vi "APU + Event Timing v6 four shots.vi"() -> ()   [LabVIEW 2015]
uses:
  IP Source/APU/Input.ctl
  IP Source/APU/Output.ctl
  IP Source/APU/Settings.ctl
  IP Source/ECU Event/Timing/Capture Output.ctl
  IP Source/ECU Event/Timing/Measure Settings.ctl
  IP Source/Version Token.ctl
  IP Source/ECU Event/Timing/Measure Output.ctl
  IP Source/APU/Shared Settings.ctl
  <vilib>/Platform/TimedLoop/XDataNode/timing_clust.ctl
  <vilib>/Platform/TimedLoop/XDataNode/nitl_modes.ctl
  <vilib>/Platform/TimedLoop/XDataNode/wakeup.ctl
  IP Source/ECU Event/Timing/Capture Settings.ctl
  <vilib>/rvi/Emulation/niFpgaSctlEmulationGetInTimedLoop.vi
  <vilib>/rvi/Emulation/niFpgaEmulationReportErrorSimple.vi
  <vilib>/rvi/Emulation/niFpgaGetClockAttributes.vi
  <vilib>/rvi/Emulation/niFpgaCriticalErrorInLSC.vi
  <vilib>/rvi/eio/common/nirviEmuTemplateMethod_errors.vi
  IP Source/ECU Event/Timing/Measure Events (40MHz).vi
  <vilib>/Platform/TimedLoop/XDataNode/XDataNode.xnode
  <vilib>/eio/EIONode/EIONode.xnode
  <vilib>/Platform/TimedLoop/XDataNode/XDNodeRunTimeDep.lvlib
  IP Source/ECU Event/Timing/ECU Event Timing.lvlib
  IP Source/APU/APU.lvlib
  IP Source/Engine Simulation Toolkit.lvlib
panel:
  in  "shared settings.my apu":T1 {"start" format="%#.15g"}
  in  "go.my apu":bool
  out "measure output.spark 4":T2
  out "measure output.spark 5":T2
  out "measure output.spark 6":T2
  out "measure output.fi 6":T2
  out "measure output.fi 5":T2
  out "measure output.fi 4":T2
  out "measure output.fi 3":T2
  out "measure output.spark 3":T2
  out "measure output.spark 2":T2
  out "measure output.spark 1":T2
  out "measure output.fi 2":T2
  out "measure output.fi 1":T2
  in  "est.version":T3
  out "Output.spark 6 shot 1":T4
  out "Output.spark 1 shot 1":T4
  out "Output.spark 2 shot 1":T4
  out "Output.spark 3 shot 1":T4
  out "Output.spark 4 shot 1":T4
  out "Output.spark 5 shot 1":T4
  out "Output.spark 6 shot 2":T4
  out "Output.spark 1 shot 2":T4
  out "Output.spark 2 shot 2":T4
  out "Output.spark 3 shot 2":T4
  out "Output.spark 4 shot 2":T4
  out "Output.spark 5 shot 2":T4
  out "Output.spark 6 shot 3":T4
  out "Output.spark 1 shot 3":T4
  out "Output.spark 2 shot 3":T4
  out "Output.spark 3 shot 3":T4
  out "Output.spark 4 shot 3":T4
  out "Output.spark 5 shot 3":T4
  out "Output.spark 6 shot 4":T4
  out "Output.spark 1 shot 4":T4
  out "Output.spark 2 shot 4":T4
  out "Output.spark 3 shot 4":T4
  out "Output.spark 4 shot 4":T4
  out "Output.spark 5 shot 4":T4
  in  "Settings.spark 1":T5
  in  "Settings.spark 2":T5
  in  "Settings.spark 3":T5
  in  "Settings.spark 4":T5
  in  "Settings.spark 5":T5
  in  "Settings.spark 6":T5
  in  "Settings.fi 6":T5
  in  "Settings.fi 5":T5
  in  "Settings.fi 4":T5
  in  "Settings.fi 3":T5
  in  "Settings.fi 2":T5
  in  "Settings.fi 1":T5
  out "Output.fi 6 shot 4":T4
  out "Output.fi 1 shot 4":T4
  out "Output.fi 2 shot 4":T4
  out "Output.fi 3 shot 4":T4
  out "Output.fi 4 shot 4":T4
  out "Output.fi 5 shot 4":T4
  out "Output.fi 6 shot 3":T4
  out "Output.fi 1 shot 3":T4
  out "Output.fi 2 shot 3":T4
  out "Output.fi 3 shot 3":T4
  out "Output.fi 4 shot 3":T4
  out "Output.fi 5 shot 3":T4
  out "Output.fi 6 shot 2":T4
  out "Output.fi 1 shot 2":T4
  out "Output.fi 2 shot 2":T4
  out "Output.fi 3 shot 2":T4
  out "Output.fi 4 shot 2":T4
  out "Output.fi 5 shot 2":T4
  out "Output.fi 5 shot 1":T4
  out "Output.fi 4 shot 1":T4
  out "Output.fi 3 shot 1":T4
  out "Output.fi 2 shot 1":T4
  out "Output.fi 1 shot 1":T4
  out "Output.fi 6 shot 1":T4
  in  "Settings.my apu":T6 caption="settings"
  out "Output.my apu":T7 caption="output"
  in  "Input.my apu":T8={"desired speed"=0.0, "reset"=TRUE} caption="input"
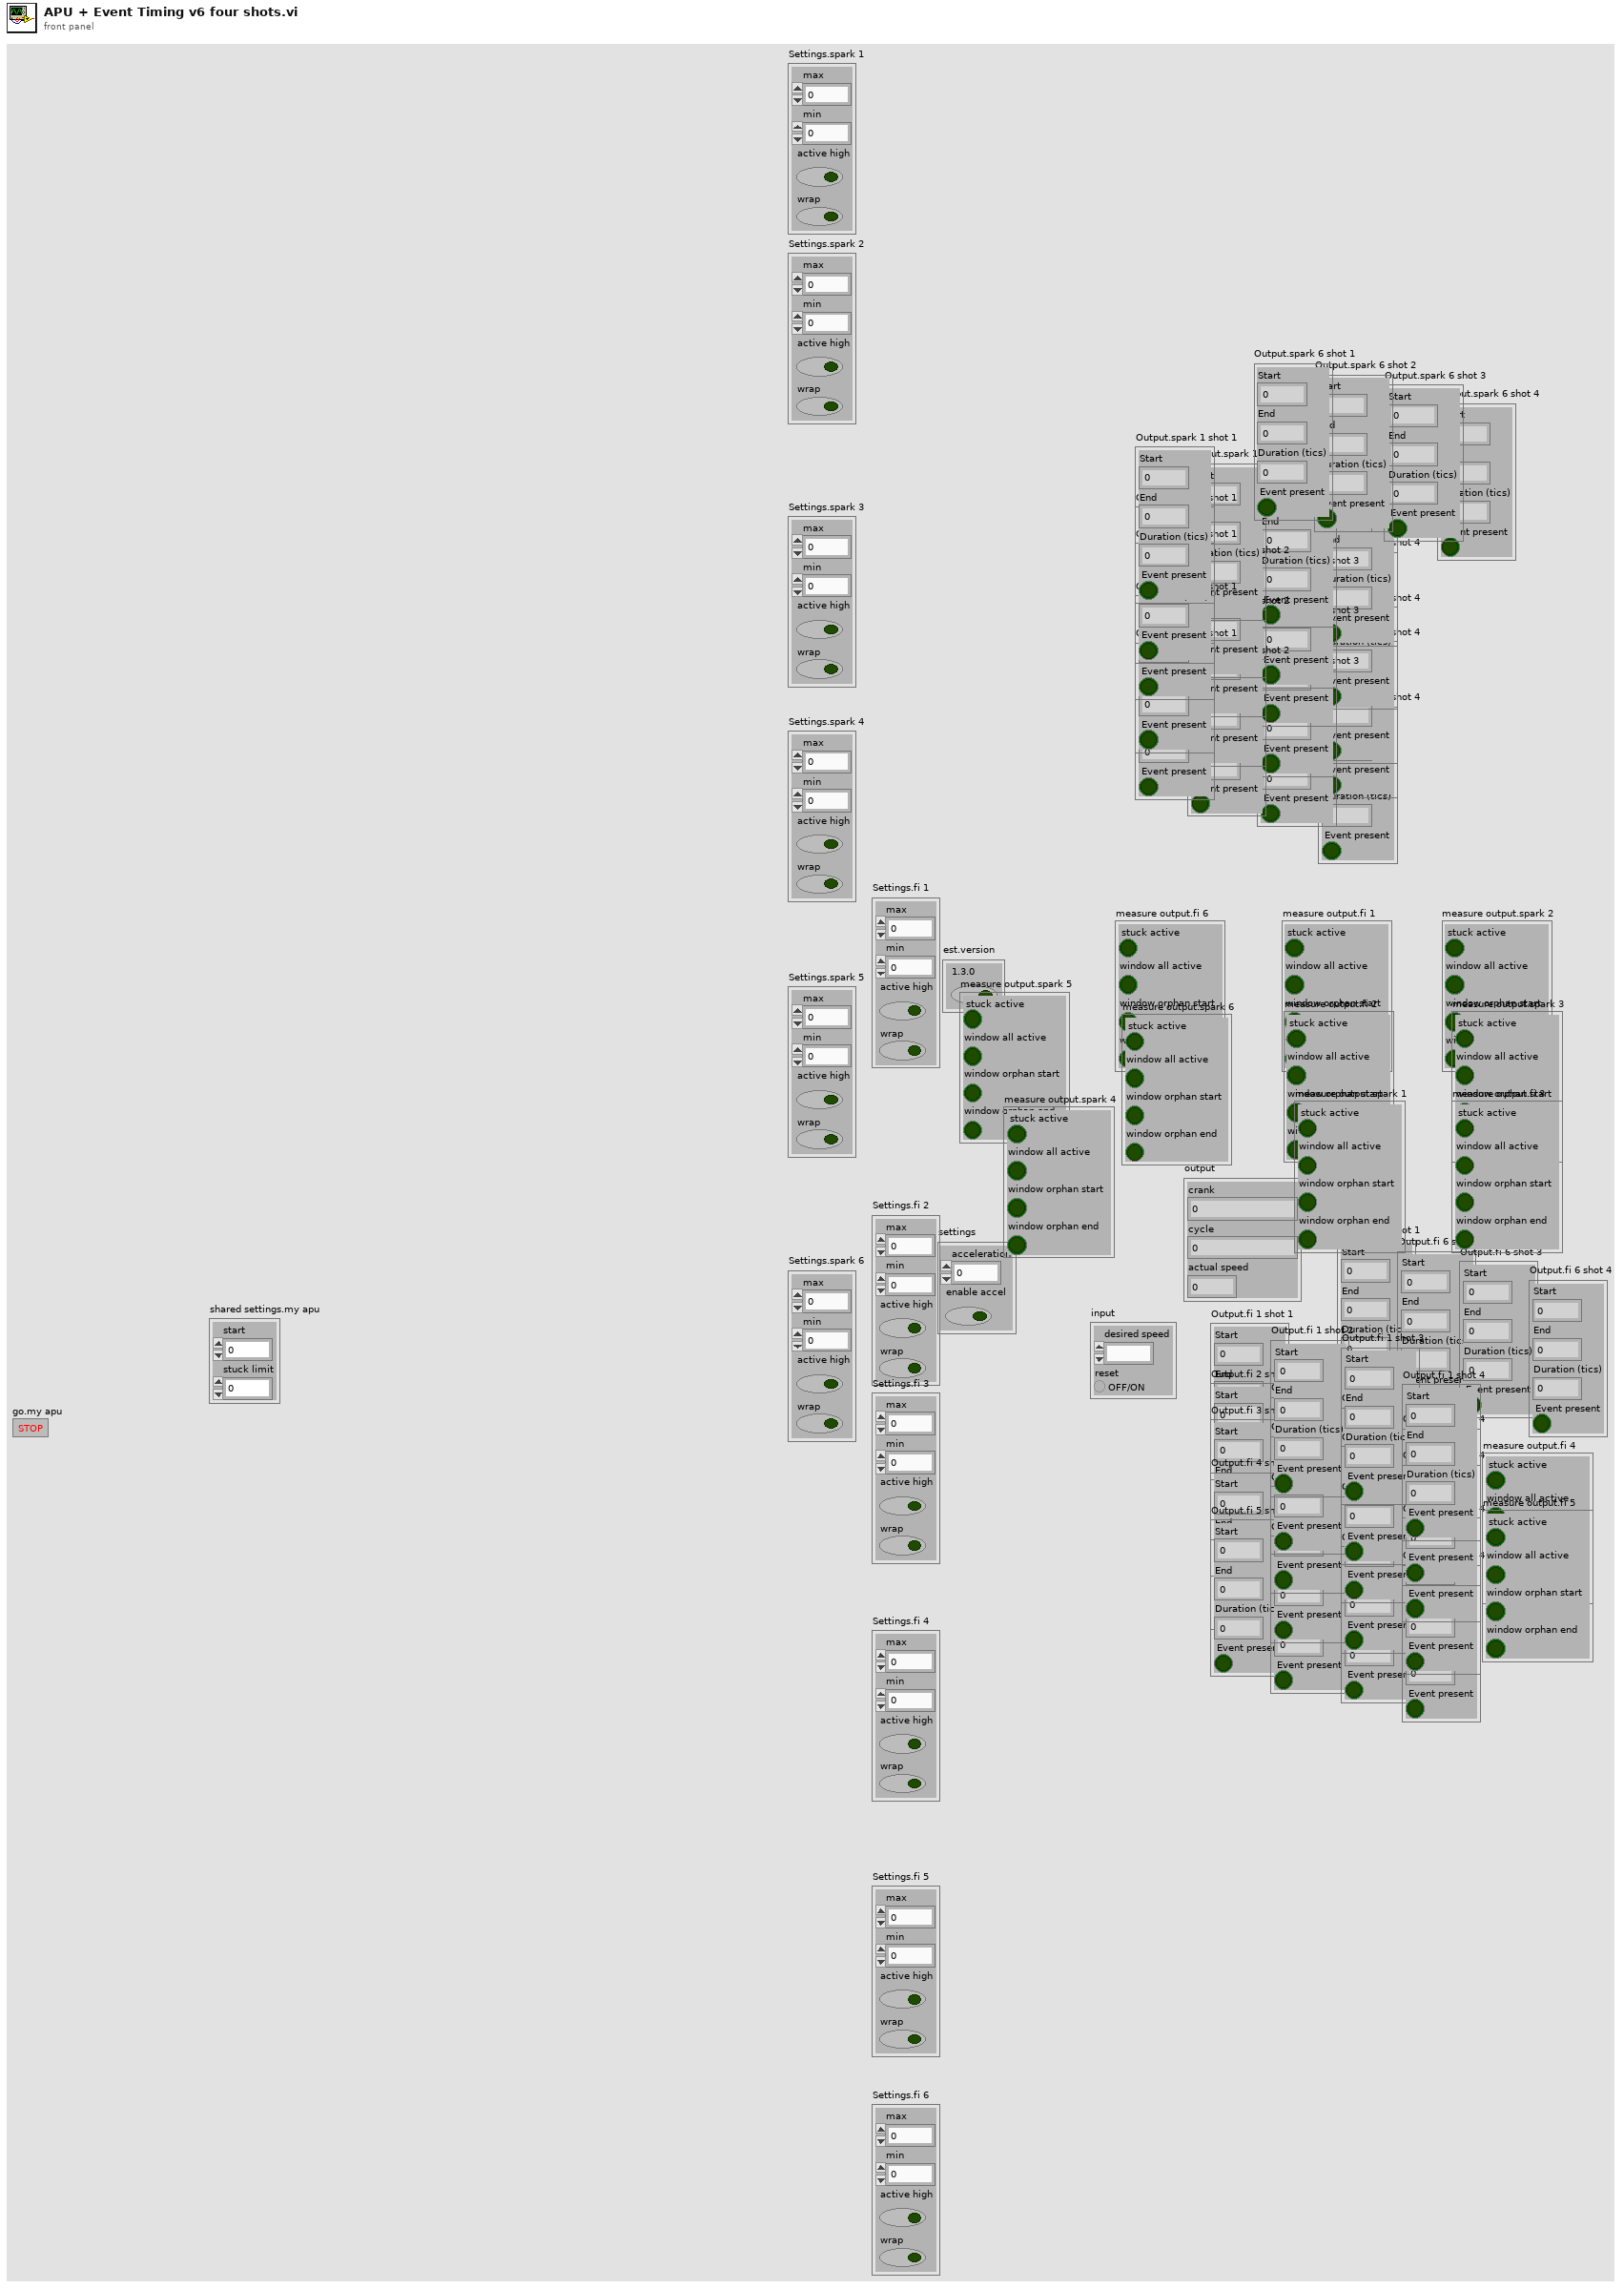
[diagram p1: front panel]
types:
  T1 = typedef "Engine Simulation Toolkit.lvlib/APU.lvlib/Shared Settings.ctl" = cluster{"start":fxp<+,17,17>, "stuck limit":fxp<+,18,18>}
  T2 = typedef "Engine Simulation Toolkit.lvlib/ECU Event Timing.lvlib/Measure Output.ctl" = cluster{"stuck active":bool, "window all active":bool, "window orphan start":bool, "window orphan end":bool}
  T3 = typedef "Engine Simulation Toolkit.lvlib/Version Token.ctl" = cluster{"1.3.0":bool}
  T4 = typedef "Engine Simulation Toolkit.lvlib/ECU Event Timing.lvlib/Capture Output.ctl" = cluster{"Start":u16, "End":u16, "Duration (tics)":fxp<+,18,18>, "Event present":bool}
  T5 = typedef "Engine Simulation Toolkit.lvlib/ECU Event Timing.lvlib/Measure Settings.ctl" = cluster{"max":u16, "min":u16, "active high":bool, "wrap":bool}
  T6 = typedef "Engine Simulation Toolkit.lvlib/APU.lvlib/Settings.ctl" = cluster{"acceleration":fxp<+,18,-20>, "enable accel":bool}
  T7 = typedef "Engine Simulation Toolkit.lvlib/APU.lvlib/Output.ctl" = cluster{"crank":u16, "cycle":u16, "actual speed":fxp<+/-,23,2>}
  T8 = typedef "Engine Simulation Toolkit.lvlib/APU.lvlib/Input.ctl" = cluster{"desired speed":fxp<+/-,23,2>, "reset":bool}
  T9 = typedef "XDNodeRunTimeDep.lvlib/timing_clust.ctl" = cluster{"Expected End [f-1]":u64, "Actual End [f-1]":u64, "Finished Late? [f-1]":bool, "Expected End [i-1]":u64, "Actual End [i-1]":u64, "Finished Late? [i-1]":bool, "Expected Start [i]":u64, "Actual Start [i]":u64, "Expected Start [f]":u64, "Actual Start [f]":u64, "Source Name":string, "Structure Name":string, "Period":i64, "Deadline":i64, "Offset":i64, "Start":i64, "Priority":i32, "Timeout":i32, "Mode":T10, "Wakeup Reason":T11, "Error":errorcluster, "Source Type":string, "Secondary Source Type":string, "Global End Time":u64, "Global Start Time":u64, "Frame Duration":u64, "Iteration Duration":u64, "Assigned CPU":i32, "I/O Scan Engine Mode":u32}
  T10 = typedef "XDNodeRunTimeDep.lvlib/nitl_modes.ctl" = enum32{"No Change", "Process missed periods, maintain original phase", "Discard missed periods, maintain original phase", "Process missed periods, ignore original phase", "Discard missed periods, ignore original phase"}
  T11 = typedef "XDNodeRunTimeDep.lvlib/wakeup.ctl" = enum32{"Normal", "Aborted", "Asynchronous wakeup", "Timing source error", "Timed loop error", "Timeout"}
  T12 = typedef "Engine Simulation Toolkit.lvlib/APU.lvlib/Register Bus.ctl" = cluster{"Speed":refnum<k21>, "Crank Angle":refnum<k21>, "Cycle Angle":refnum<k21>, "Crank Count":refnum<k21>, "Cycle Count":refnum<k21>, "1.25 MHz Counter":refnum<k21>, "Crank Rollover":refnum<k21>, "Cycle Rollover":refnum<k21>, "shared settings":T1}
  T13 = typedef "Engine Simulation Toolkit.lvlib/ECU Event Timing.lvlib/Capture Settings.ctl" = u8
  T14 = typedef "Engine Simulation Toolkit.lvlib/ECU Event Timing.lvlib/Measured Data.ctl" = cluster{"start":u16, "end":u16, "duration (tics)":fxp<+,18,18>, "window end":bool, "window begin":bool, "pulse end":bool, "pulse #":u8}
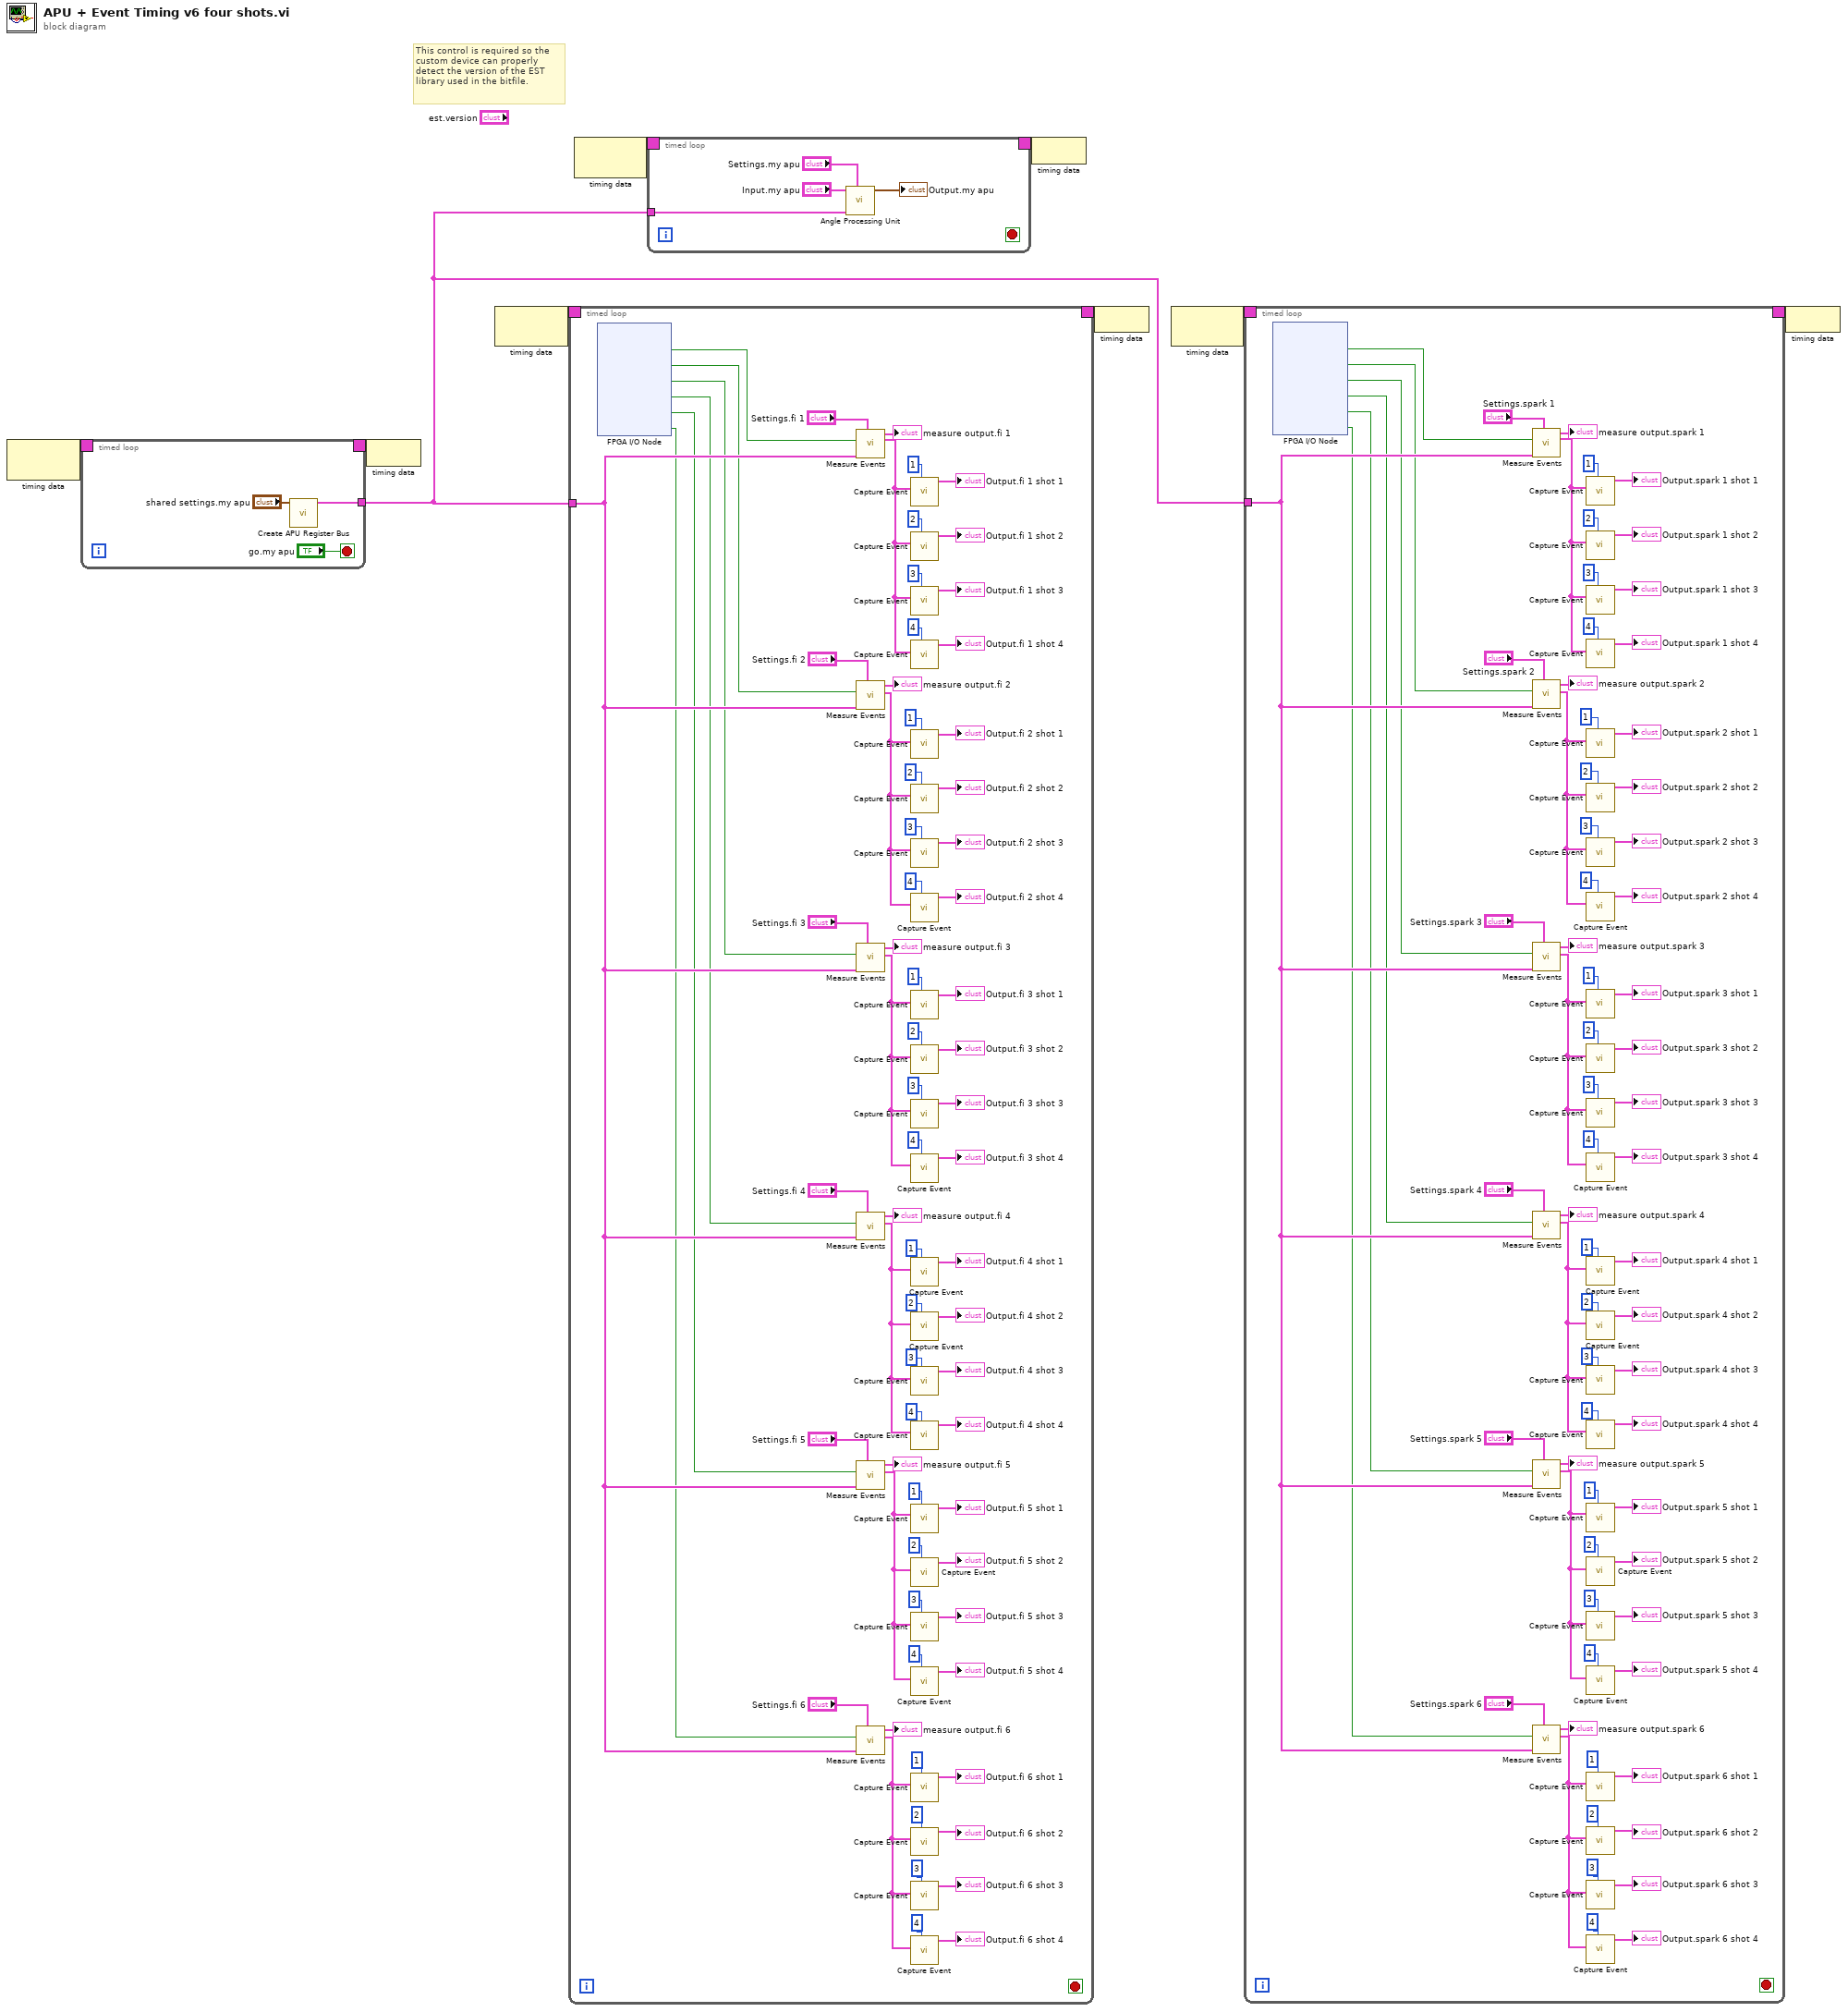
[diagram p0: block diagram]
diagram:
  # "This control is required so the custom device can properly detect the version of the EST library used in the bitfile."
  n1 = node-c288() -> (w3:T9)  [unwired: 1 in]
  n2 = timed-loop {
    timing: w3 -> [_]
    timing-out: [_] -> w2
    tunnel: [w12] -> w1
    stop <- "go.my apu" stop-if-true
    n3 = call "Create APU Register Bus.vi"("shared settings.<user name>"="shared settings.my apu") -> ("register bus"=w12:T12)  [unwired: 10 in]
  }
  n4 = node-c288(w2) -> ()
  n5 = node-c288() -> (w7:T9)  [unwired: 1 in]
  n6 = timed-loop {
    timing: w7 -> [_]
    timing-out: [_] -> w6
    tunnel: w1 -> [w63]
    stop <- _ stop-if-true
    n7 = xnode "FPGA I/O Node"() -> ("DIO0_0"=w56:bool, "DIO1_0"=w36:bool, "DIO2_0"=w35:bool, "DIO3_0"=w34:bool, "DIO4_0"=w22:bool, "DIO5_0"=w21:bool)  [unwired: 6 in, 6 out]
    n8 = call-poly "Measure Events.vi"("settings.<user name>"="Settings.fi 1", "register bus"=w63, "event"=w56) -> ("measured data"=w57:T14, "status.<user name>"=→"measure output.fi 1":T2)  [unwired: 7 in]
    n9 = call-poly "Measure Events.vi"("settings.<user name>"="Settings.fi 2", "register bus"=w63, "event"=w36) -> ("measured data"=w37:T14, "status.<user name>"=→"measure output.fi 2":T2)  [unwired: 7 in]
    n10 = call-poly "Measure Events.vi"("settings.<user name>"="Settings.fi 3", "register bus"=w63, "event"=w35) -> ("measured data"=w29:T14, "status.<user name>"=→"measure output.fi 3":T2)  [unwired: 7 in]
    n11 = call-poly "Measure Events.vi"("settings.<user name>"="Settings.fi 4", "register bus"=w63, "event"=w34) -> ("measured data"=w24:T14, "status.<user name>"=→"measure output.fi 4":T2)  [unwired: 7 in]
    n12 = call-poly "Measure Events.vi"("settings.<user name>"="Settings.fi 5", "register bus"=w63, "event"=w22) -> ("measured data"=w23:T14, "status.<user name>"=→"measure output.fi 5":T2)  [unwired: 7 in]
    n13 = call-poly "Measure Events.vi"("settings.<user name>"="Settings.fi 6", "register bus"=w63, "event"=w21) -> ("measured data"=w46:T14, "status.<user name>"=→"measure output.fi 6":T2)  [unwired: 7 in]
    n14 = call "Capture Event.vi"("event # to capture"=T13 1 ("Settings.fi 1 shot 1"), "measured data"=w57) -> ("capture.<user name>"=→"Output.fi 1 shot 1":T4)  [unwired: 9 in]
    n15 = call "Capture Event.vi"("event # to capture"=T13 2 ("Settings.fi 1 shot 2"), "measured data"=w57) -> ("capture.<user name>"=→"Output.fi 1 shot 2":T4)  [unwired: 9 in]
    n16 = call "Capture Event.vi"("event # to capture"=T13 3 ("Settings.fi 1 shot 3"), "measured data"=w57) -> ("capture.<user name>"=→"Output.fi 1 shot 3":T4)  [unwired: 9 in]
    n17 = call "Capture Event.vi"("event # to capture"=T13 4 ("Settings.fi 1 shot 4"), "measured data"=w57) -> ("capture.<user name>"=→"Output.fi 1 shot 4":T4)  [unwired: 9 in]
    n18 = call "Capture Event.vi"("event # to capture"=T13 1 ("Settings.fi 1 shot 1"), "measured data"=w37) -> ("capture.<user name>"=→"Output.fi 2 shot 1":T4)  [unwired: 9 in]
    n19 = call "Capture Event.vi"("event # to capture"=T13 2 ("Settings.fi 1 shot 2"), "measured data"=w37) -> ("capture.<user name>"=→"Output.fi 2 shot 2":T4)  [unwired: 9 in]
    n20 = call "Capture Event.vi"("event # to capture"=T13 3 ("Settings.fi 1 shot 3"), "measured data"=w37) -> ("capture.<user name>"=→"Output.fi 2 shot 3":T4)  [unwired: 9 in]
    n21 = call "Capture Event.vi"("event # to capture"=T13 4 ("Settings.fi 1 shot 4"), "measured data"=w37) -> ("capture.<user name>"=→"Output.fi 2 shot 4":T4)  [unwired: 9 in]
    n22 = call "Capture Event.vi"("event # to capture"=T13 1 ("Settings.fi 1 shot 1"), "measured data"=w29) -> ("capture.<user name>"=→"Output.fi 3 shot 1":T4)  [unwired: 9 in]
    n23 = call "Capture Event.vi"("event # to capture"=T13 2 ("Settings.fi 1 shot 2"), "measured data"=w29) -> ("capture.<user name>"=→"Output.fi 3 shot 2":T4)  [unwired: 9 in]
    n24 = call "Capture Event.vi"("event # to capture"=T13 3 ("Settings.fi 1 shot 3"), "measured data"=w29) -> ("capture.<user name>"=→"Output.fi 3 shot 3":T4)  [unwired: 9 in]
    n25 = call "Capture Event.vi"("event # to capture"=T13 4 ("Settings.fi 1 shot 4"), "measured data"=w29) -> ("capture.<user name>"=→"Output.fi 3 shot 4":T4)  [unwired: 9 in]
    n26 = call "Capture Event.vi"("event # to capture"=T13 1 ("Settings.fi 1 shot 1"), "measured data"=w24) -> ("capture.<user name>"=→"Output.fi 4 shot 1":T4)  [unwired: 9 in]
    n27 = call "Capture Event.vi"("event # to capture"=T13 2 ("Settings.fi 1 shot 2"), "measured data"=w24) -> ("capture.<user name>"=→"Output.fi 4 shot 2":T4)  [unwired: 9 in]
    n28 = call "Capture Event.vi"("event # to capture"=T13 3 ("Settings.fi 1 shot 3"), "measured data"=w24) -> ("capture.<user name>"=→"Output.fi 4 shot 3":T4)  [unwired: 9 in]
    n29 = call "Capture Event.vi"("event # to capture"=T13 4 ("Settings.fi 1 shot 4"), "measured data"=w24) -> ("capture.<user name>"=→"Output.fi 4 shot 4":T4)  [unwired: 9 in]
    n30 = call "Capture Event.vi"("event # to capture"=T13 1 ("Settings.fi 1 shot 1"), "measured data"=w23) -> ("capture.<user name>"=→"Output.fi 5 shot 1":T4)  [unwired: 9 in]
    n31 = call "Capture Event.vi"("event # to capture"=T13 2 ("Settings.fi 1 shot 2"), "measured data"=w23) -> ("capture.<user name>"=→"Output.fi 5 shot 2":T4)  [unwired: 9 in]
    n32 = call "Capture Event.vi"("event # to capture"=T13 3 ("Settings.fi 1 shot 3"), "measured data"=w23) -> ("capture.<user name>"=→"Output.fi 5 shot 3":T4)  [unwired: 9 in]
    n33 = call "Capture Event.vi"("event # to capture"=T13 4 ("Settings.fi 1 shot 4"), "measured data"=w23) -> ("capture.<user name>"=→"Output.fi 5 shot 4":T4)  [unwired: 9 in]
    n34 = call "Capture Event.vi"("event # to capture"=T13 1 ("Settings.fi 1 shot 1"), "measured data"=w46) -> ("capture.<user name>"=→"Output.fi 6 shot 1":T4)  [unwired: 9 in]
    n35 = call "Capture Event.vi"("event # to capture"=T13 2 ("Settings.fi 1 shot 2"), "measured data"=w46) -> ("capture.<user name>"=→"Output.fi 6 shot 2":T4)  [unwired: 9 in]
    n36 = call "Capture Event.vi"("event # to capture"=T13 3 ("Settings.fi 1 shot 3"), "measured data"=w46) -> ("capture.<user name>"=→"Output.fi 6 shot 3":T4)  [unwired: 9 in]
    n37 = call "Capture Event.vi"("event # to capture"=T13 4 ("Settings.fi 1 shot 4"), "measured data"=w46) -> ("capture.<user name>"=→"Output.fi 6 shot 4":T4)  [unwired: 9 in]
  }
  n38 = node-c288() -> (w9:T9)  [unwired: 1 in]
  n39 = timed-loop {
    timing: w9 -> [_]
    timing-out: [_] -> w8
    tunnel: w1 -> [w90]
    stop <- _ stop-if-true
    n40 = call "Angle Processing Unit.vi"("settings.<user name>"="Settings.my apu", "register bus"=w90, "input.<user name>"="Input.my apu") -> ("output.<user name>"=→"Output.my apu":T7)  [unwired: 8 in]
  }
  n41 = node-c288(w8) -> ()
  n42 = node-c288(w6) -> ()
  n43 = node-c288() -> (w5:T9)  [unwired: 1 in]
  n44 = timed-loop {
    timing: w5 -> [_]
    timing-out: [_] -> w4
    tunnel: w1 -> [w144]
    stop <- _ stop-if-true
    n45 = xnode "FPGA I/O Node"() -> ("DIO0_1"=w137:bool, "DIO1_1"=w117:bool, "DIO2_1"=w116:bool, "DIO3_1"=w115:bool, "DIO4_1"=w103:bool, "DIO5_1"=w102:bool)  [unwired: 6 in, 6 out]
    n46 = call-poly "Measure Events.vi"("settings.<user name>"="Settings.spark 1", "register bus"=w144, "event"=w137) -> ("measured data"=w138:T14, "status.<user name>"=→"measure output.spark 1":T2)  [unwired: 7 in]
    n47 = call-poly "Measure Events.vi"("settings.<user name>"="Settings.spark 2", "register bus"=w144, "event"=w117) -> ("measured data"=w118:T14, "status.<user name>"=→"measure output.spark 2":T2)  [unwired: 7 in]
    n48 = call-poly "Measure Events.vi"("settings.<user name>"="Settings.spark 3", "register bus"=w144, "event"=w116) -> ("measured data"=w110:T14, "status.<user name>"=→"measure output.spark 3":T2)  [unwired: 7 in]
    n49 = call-poly "Measure Events.vi"("settings.<user name>"="Settings.spark 4", "register bus"=w144, "event"=w115) -> ("measured data"=w105:T14, "status.<user name>"=→"measure output.spark 4":T2)  [unwired: 7 in]
    n50 = call-poly "Measure Events.vi"("settings.<user name>"="Settings.spark 5", "register bus"=w144, "event"=w103) -> ("measured data"=w104:T14, "status.<user name>"=→"measure output.spark 5":T2)  [unwired: 7 in]
    n51 = call-poly "Measure Events.vi"("settings.<user name>"="Settings.spark 6", "register bus"=w144, "event"=w102) -> ("measured data"=w127:T14, "status.<user name>"=→"measure output.spark 6":T2)  [unwired: 7 in]
    n52 = call "Capture Event.vi"("event # to capture"=T13 1 ("Settings.spark 1 shot 1"), "measured data"=w138) -> ("capture.<user name>"=→"Output.spark 1 shot 1":T4)  [unwired: 9 in]
    n53 = call "Capture Event.vi"("event # to capture"=T13 2 ("Settings.spark 1 shot 2"), "measured data"=w138) -> ("capture.<user name>"=→"Output.spark 1 shot 2":T4)  [unwired: 9 in]
    n54 = call "Capture Event.vi"("event # to capture"=T13 3 ("Settings.spark 1 shot 3"), "measured data"=w138) -> ("capture.<user name>"=→"Output.spark 1 shot 3":T4)  [unwired: 9 in]
    n55 = call "Capture Event.vi"("event # to capture"=T13 4 ("Settings.spark 1 shot 4"), "measured data"=w138) -> ("capture.<user name>"=→"Output.spark 1 shot 4":T4)  [unwired: 9 in]
    n56 = call "Capture Event.vi"("event # to capture"=T13 1 ("Settings.spark 1 shot 1"), "measured data"=w118) -> ("capture.<user name>"=→"Output.spark 2 shot 1":T4)  [unwired: 9 in]
    n57 = call "Capture Event.vi"("event # to capture"=T13 2 ("Settings.spark 1 shot 2"), "measured data"=w118) -> ("capture.<user name>"=→"Output.spark 2 shot 2":T4)  [unwired: 9 in]
    n58 = call "Capture Event.vi"("event # to capture"=T13 3 ("Settings.spark 1 shot 3"), "measured data"=w118) -> ("capture.<user name>"=→"Output.spark 2 shot 3":T4)  [unwired: 9 in]
    n59 = call "Capture Event.vi"("event # to capture"=T13 4 ("Settings.spark 1 shot 4"), "measured data"=w118) -> ("capture.<user name>"=→"Output.spark 2 shot 4":T4)  [unwired: 9 in]
    n60 = call "Capture Event.vi"("event # to capture"=T13 1 ("Settings.spark 1 shot 1"), "measured data"=w110) -> ("capture.<user name>"=→"Output.spark 3 shot 1":T4)  [unwired: 9 in]
    n61 = call "Capture Event.vi"("event # to capture"=T13 2 ("Settings.spark 1 shot 2"), "measured data"=w110) -> ("capture.<user name>"=→"Output.spark 3 shot 2":T4)  [unwired: 9 in]
    n62 = call "Capture Event.vi"("event # to capture"=T13 3 ("Settings.spark 1 shot 3"), "measured data"=w110) -> ("capture.<user name>"=→"Output.spark 3 shot 3":T4)  [unwired: 9 in]
    n63 = call "Capture Event.vi"("event # to capture"=T13 4 ("Settings.spark 1 shot 4"), "measured data"=w110) -> ("capture.<user name>"=→"Output.spark 3 shot 4":T4)  [unwired: 9 in]
    n64 = call "Capture Event.vi"("event # to capture"=T13 1 ("Settings.spark 1 shot 1"), "measured data"=w105) -> ("capture.<user name>"=→"Output.spark 4 shot 1":T4)  [unwired: 9 in]
    n65 = call "Capture Event.vi"("event # to capture"=T13 2 ("Settings.spark 1 shot 2"), "measured data"=w105) -> ("capture.<user name>"=→"Output.spark 4 shot 2":T4)  [unwired: 9 in]
    n66 = call "Capture Event.vi"("event # to capture"=T13 3 ("Settings.spark 1 shot 3"), "measured data"=w105) -> ("capture.<user name>"=→"Output.spark 4 shot 3":T4)  [unwired: 9 in]
    n67 = call "Capture Event.vi"("event # to capture"=T13 4 ("Settings.spark 1 shot 4"), "measured data"=w105) -> ("capture.<user name>"=→"Output.spark 4 shot 4":T4)  [unwired: 9 in]
    n68 = call "Capture Event.vi"("event # to capture"=T13 1 ("Settings.spark 1 shot 1"), "measured data"=w104) -> ("capture.<user name>"=→"Output.spark 5 shot 1":T4)  [unwired: 9 in]
    n69 = call "Capture Event.vi"("event # to capture"=T13 2 ("Settings.spark 1 shot 2"), "measured data"=w104) -> ("capture.<user name>"=→"Output.spark 5 shot 2":T4)  [unwired: 9 in]
    n70 = call "Capture Event.vi"("event # to capture"=T13 3 ("Settings.spark 1 shot 3"), "measured data"=w104) -> ("capture.<user name>"=→"Output.spark 5 shot 3":T4)  [unwired: 9 in]
    n71 = call "Capture Event.vi"("event # to capture"=T13 4 ("Settings.spark 1 shot 4"), "measured data"=w104) -> ("capture.<user name>"=→"Output.spark 5 shot 4":T4)  [unwired: 9 in]
    n72 = call "Capture Event.vi"("event # to capture"=T13 1 ("Settings.spark 1 shot 1"), "measured data"=w127) -> ("capture.<user name>"=→"Output.spark 6 shot 1":T4)  [unwired: 9 in]
    n73 = call "Capture Event.vi"("event # to capture"=T13 2 ("Settings.spark 1 shot 2"), "measured data"=w127) -> ("capture.<user name>"=→"Output.spark 6 shot 2":T4)  [unwired: 9 in]
    n74 = call "Capture Event.vi"("event # to capture"=T13 3 ("Settings.spark 1 shot 3"), "measured data"=w127) -> ("capture.<user name>"=→"Output.spark 6 shot 3":T4)  [unwired: 9 in]
    n75 = call "Capture Event.vi"("event # to capture"=T13 4 ("Settings.spark 1 shot 4"), "measured data"=w127) -> ("capture.<user name>"=→"Output.spark 6 shot 4":T4)  [unwired: 9 in]
  }
  n76 = node-c288(w4) -> ()
